vi "LVClass_Pupil Set Data.vi"(0 "Pupil in":refnum<class "Pupil.lvclass">, 5 "Data":u8[][](array[numeric]), 11 "error in (no error)":errorcluster) -> (4 "Pupil out":refnum<class "Pupil.lvclass">, 15 "error out":errorcluster)   [LabVIEW 2020, in "Pupil.lvclass"]
doc: "Set Pupil buffer.\n\n--------------------------------------------------------------------------------\n\n<B>PupilIn </B> : Pupil object.\n<B>PupilOut </B> : Pupil object.\n<B>data </B> : Pupil buffer to set.\n<B>ErrorIn </B> : Error\n<B>ErrorOut </B> : Error\n\n--------------------------------------------------------------------------------"
uses:
  Pupil.lvclass
  Pupil.lvclass/Pupil.ctl
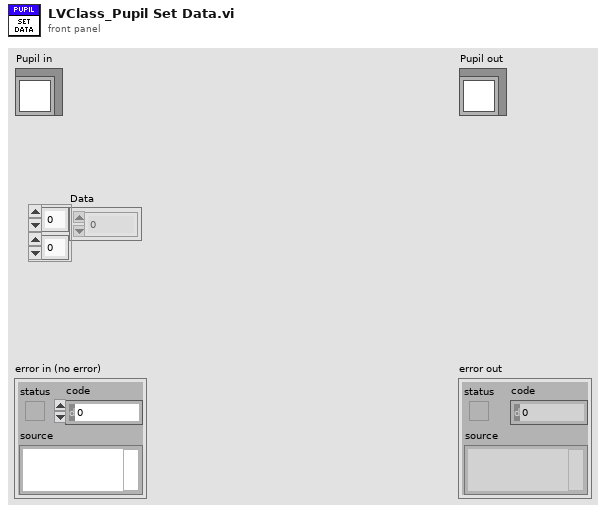
[diagram p1: front panel]
types:
  T1 = typedef "General dimensions definition.ctl" = cluster{"Size":T2, "Step":T3}
  T2 = typedef "Point2D.ctl" = cluster{"X":u32, "Y":u32}
  T3 = typedef "Point2Df.ctl" = cluster{"X":sgl, "Y":sgl}
  T4 = typedef "ClassID.ctl" = i64
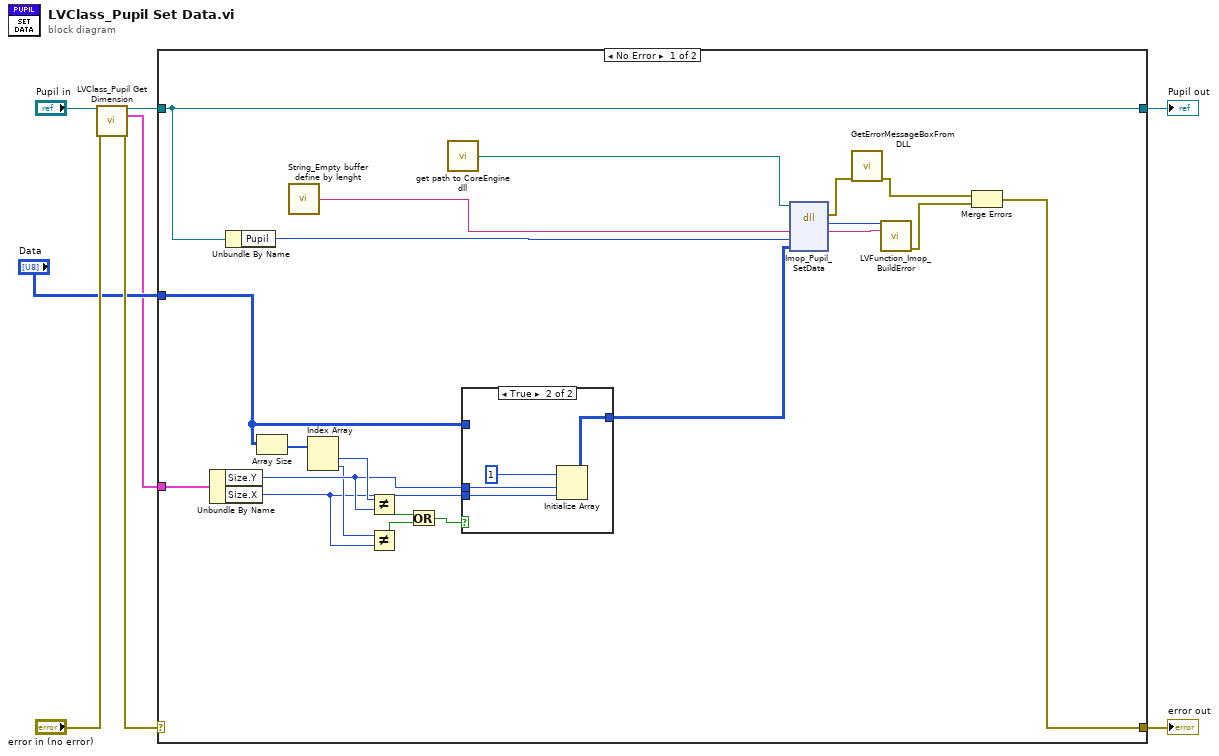
[diagram p0: block diagram]
diagram:
  n1 = call "LVClass_Pupil Get Dimension.vi"("Pupil in"="Pupil in", "error in (no error)"="error in (no error)") -> ("Pupil out"=w3:refnum<class "Pupil.lvclass">, "Dimension"=w1:T1, "error out"=w5:errorcluster)  [unwired: 11 in]
  n2 = case shown="No Error" w5 {
    selector: w5 -> [_ w36]
    tunnel: [w20 w36] -> w8
    tunnel: [w24 w35] -> w7
    tunnel: w3 -> [w24 w35]
    tunnel: "Data" -> [w10 _]
    tunnel: w1 -> [w11 _]
    frame No Error {
      n3 = Unbundle By Name(w11) -> ("Size.Y"=w17:u32, "Size.X"=w15:u32)
      n4 = Unbundle By Name(w24) -> ("Pupil"=w23:T4)
      n5 = Array Size(array=w10) -> (size(s)=w19:i32[])
      n6 = call "String_Empty buffer define by lenght.vi"() -> ("Empty buffer"=w29:string)  [unwired: 1 in]
      n7 = Index Array(array=w19) -> (element #1=w18:i32, element #2=w16:i32)  [unwired: 2 in]
      n8 = Not Equal?(x=w18, y=w17) -> (x != y?=w14:bool)
      n9 = Not Equal?(x=w16, y=w15) -> (x != y?=w13:bool)
      n10 = Or(x=w14, y=w13) -> (x .or. y?=w12:bool)
      n11 = call "get path to CoreEngine dll.vi"() -> ("path to wavekit library"=w26:path)  [unwired: 14 in, 1 out]
      n12 = case shown="True" w12 {
        tunnel: [w30 w32] -> w9
        tunnel: w17 -> [_ w34]
        tunnel: w15 -> [_ w33]
        tunnel: w10 -> [w30 _]
        frame False {
        }
        frame True {
          n13 = Initialize Array(u8 1, w34, w33) -> (w32:u8[][])
        }
      }
      n14 = dll-call lib="D:/2_trunk/Soft_haso/ImOpCoreEngine4_LV2011/DLLs/ImopEngine4_vc100.dll" fn="Imop_Pupil_SetData"(path in=w26, "message"=w29, "objet"=w23, "Data"=w9) -> (error out=w25:errorcluster, "return type"=w27:i32, "message"=w28:string)  [unwired: 4 in, 1 out]
      n15 = call "GetErrorMessageBoxFromDLL.vi"("error IN"=w25) -> ("error OUT"=w22:errorcluster)  [unwired: 10 in]
      n16 = call "LVFunction_Imop_BuildError.vi"("code"=w27, "String to Prepend to source (\"\")"=w28) -> ("error out"=w21:errorcluster)  [unwired: 13 in]
      n17 = Merge Errors(w22, w21) -> (w20:errorcluster)
    }
    frame Error {
    }
  }
  "error out" <- w8
  "Pupil out" <- w7
